vi "06记录拆表格.vi"(1 "16类（被收）":string[](array[string])) -> (15 "拆分显示（主页）":string[][](array[string]))   [LabVIEW 2019]
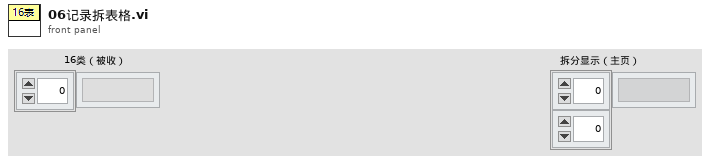
[diagram p1: front panel]
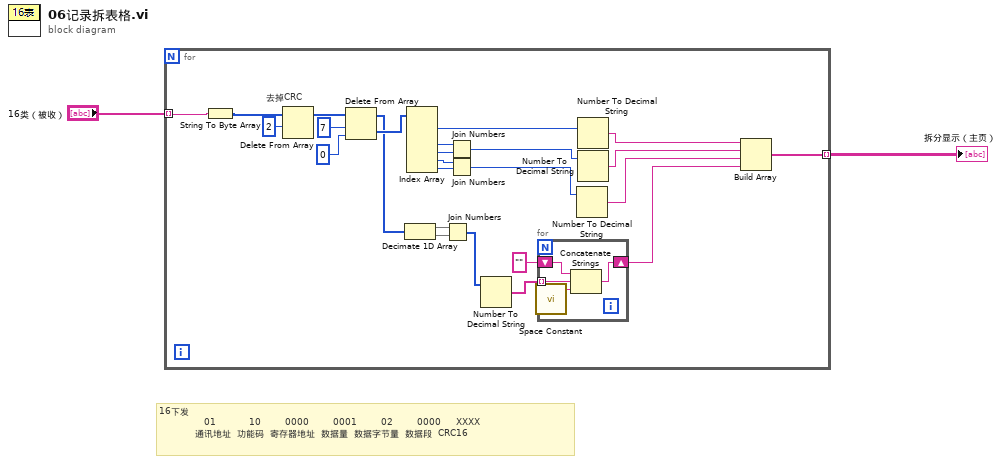
[diagram p0: block diagram]
diagram:
  # "16下发\n               01           10        0000        0001        02        0000     XXXX\n            通讯地址  功能码  寄存器地址  数据量  数据字节量  数据段  CRC16"
  n1 = for {
    tunnel: "16类（被收）" -> [w15] mode=indexing
    tunnel: [w3] -> w1 mode=indexing
    # "去掉CRC"
    n2 = String To Byte Array(string=w15) -> (unsigned byte array=w14:u8[])
    n3 = Delete From Array(array=w14, length=2 ("长度")) -> (array with subset deleted=w26:u8[])  [unwired: 1 in, 1 out]
    n4 = Delete From Array(array=w26, length=7 ("长度"), index=0 ("索引")) -> (deleted portion=w19:u8[], array with subset deleted=w13:u8[])
    n5 = Decimate 1D Array(w13) -> (w18:u8[], w12:u8[])
    n6 = Index Array(array=w19) -> (element #1=w10:u8, element #3=w21:u8, element #4=w20:u8, element #5=w23:u8, element #6=w22:u8)  [unwired: 6 in, 1 out]
    n7 = Join Numbers(hi=w18, lo=w12) -> ((hi.lo)=w11:u16[])
    n8 = Join Numbers(hi=w21, lo=w20) -> ((hi.lo)=w9:u16)
    n9 = Join Numbers(hi=w23, lo=w22) -> ((hi.lo)=w8:u16)
    n10 = Number To Decimal String(number=w11) -> (decimal integer string=w17:string[])  [unwired: 1 in]
    n11 = for {
      tunnel: w17 -> [w31] mode=indexing
      shift-right: [w29] -> w4
      shift-left: "" -> [w30]
      n12 = call <vilib>:"Space Constant.vi"() -> ("String"=w28:string)
      n13 = Concatenate Strings(w30, w31, w28) -> (w29:string)
    }
    n14 = Number To Decimal String(number=w8) -> (decimal integer string=w5:string)  [unwired: 1 in]
    n15 = Number To Decimal String(number=w10) -> (decimal integer string=w7:string)  [unwired: 1 in]
    n16 = Number To Decimal String(number=w9) -> (decimal integer string=w6:string)  [unwired: 1 in]
    n17 = Build Array(w7, w6, w5, w4) -> (w3:string[])
  }
  "拆分显示（主页）" <- w1
